vi "Measure - con-stay.vi"() -> ()   [LabVIEW 2013]
panel:
  in  "errorOutt":errorcluster
  in  "Error":bool
  in  "SetOutput":bool
  in  "NeedToSetOutput":bool
  out "Output":string
  out "SetCurrentStr":string
  out "SetVoltageStr":string
  in  "SetVoltage":dbl format="%#.3g"
  in  "SetCurrent":dbl
  in  "NeedToSetVoltage":bool
  in  "NeedToSetCurrent":bool
  in  "Active":bool
  out "connection ID":refnum<k5>
  in  "Connect":bool
  out "GetCurrent":string
  in  "Adress":string="172.16.21.19"
  out "GetVoltage":string
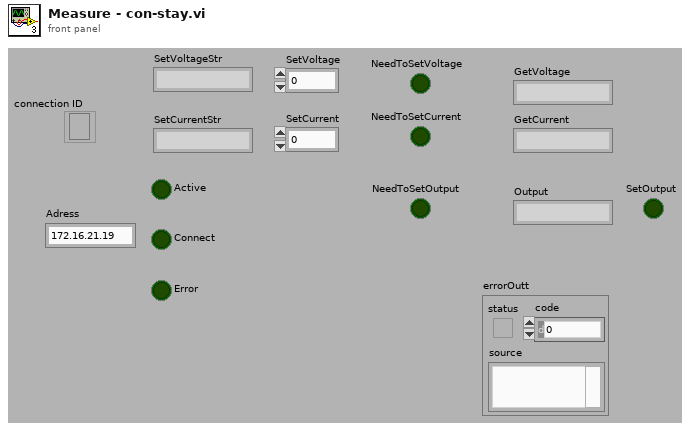
[diagram p1: front panel]
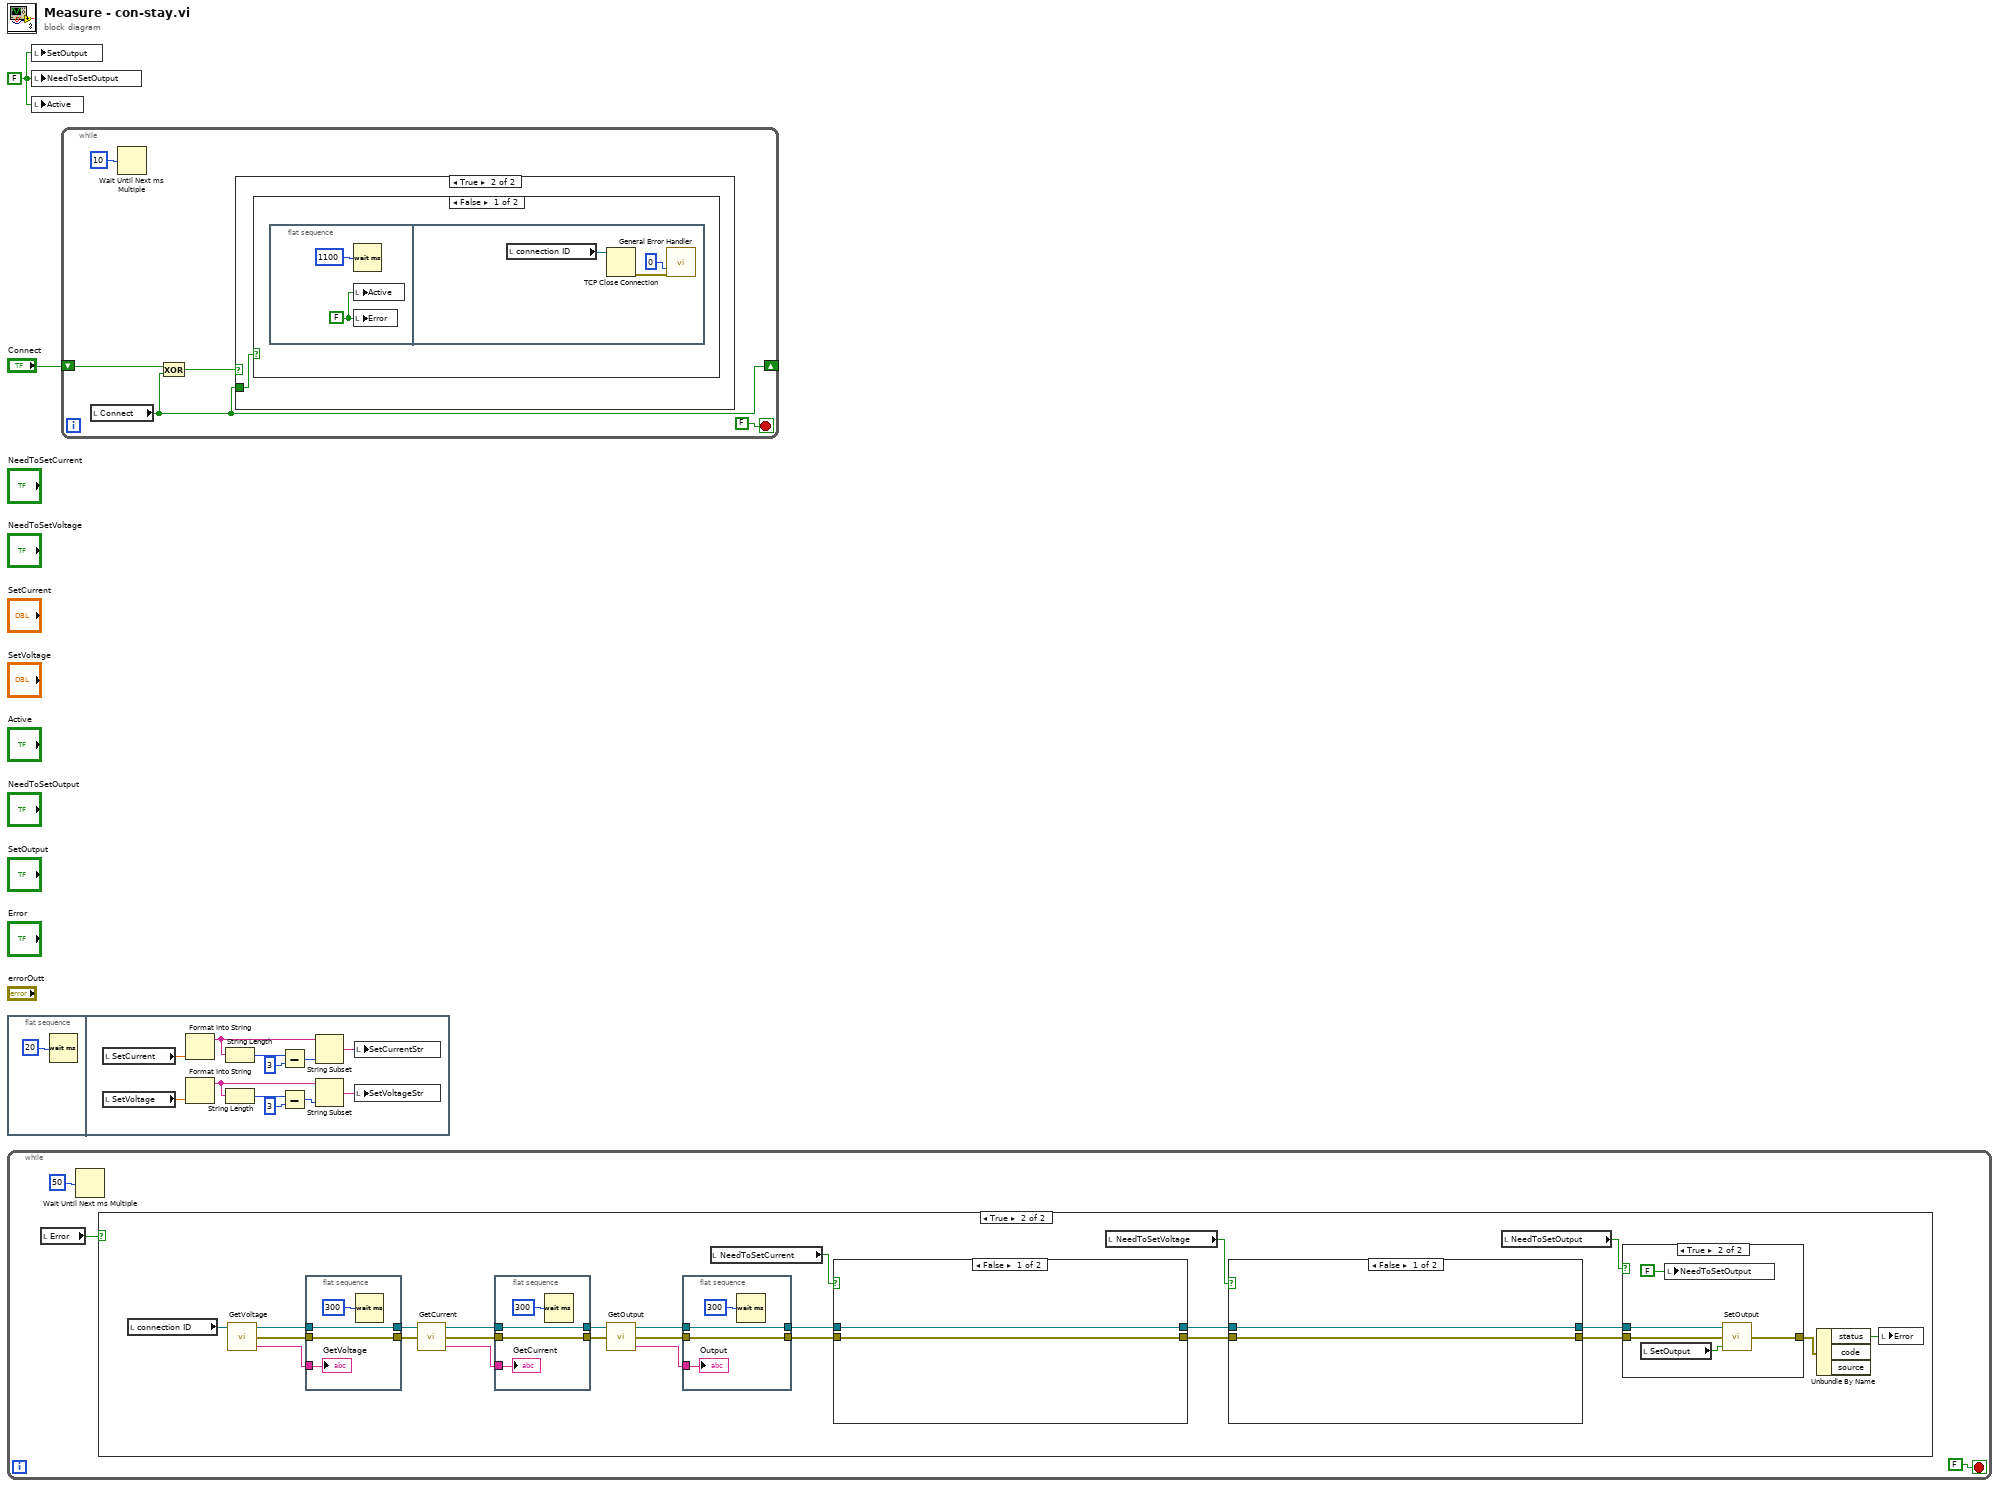
[diagram p0: block diagram]
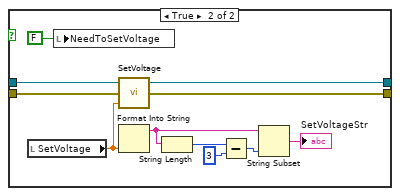
[diagram p4: hidden frame]
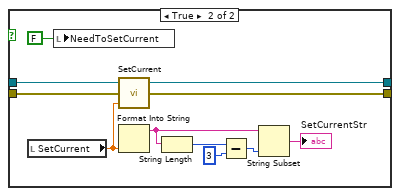
[diagram p5: hidden frame]
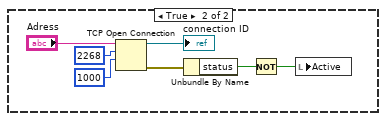
[diagram p7: hidden frame]
diagram:
  w1 = FALSE ("Active")
  n1 = flat-sequence {
    frame #0 {
      n2 = Wait (ms)(milliseconds to wait=u32 20 ("millisecond multiple")) -> ()  [unwired: 1 out]
    }
    frame #1 {
      n3 = local read "SetCurrent"() -> (w11:dbl)
      n4 = local read "SetVoltage"() -> (w10:dbl)
      n5 = Format Into String(w11) -> (resulting string=w15:string)  [unwired: 3 in, 1 out]
      n6 = Format Into String(w10) -> (resulting string=w6:string)  [unwired: 3 in, 1 out]
      n7 = String Length(string=w15) -> (length=w14:i32)
      n8 = String Length(string=w6) -> (length=w9:i32)
      n9 = Subtract(x=w14, y=3) -> (x-y=w12:i32)
      n10 = Subtract(x=w9, y=3) -> (x-y=w7:i32)
      n11 = String Subset(string=w15, length (rest)=w12) -> (substring=w4:string)  [unwired: 1 out]
      n12 = String Subset(string=w6, length (rest)=w7) -> (substring=w5:string)  [unwired: 1 out]
      n13 = local write "SetCurrentStr"(w4) -> ()
      n14 = local write "SetVoltageStr"(w5) -> ()
    }
  }
  n15 = while {
    stop <- FALSE stop-if-true
    n16 = local read "Error"() -> (w17:bool)
    n17 = Wait Until Next ms Multiple(millisecond multiple=u32 50) -> ()  [unwired: 1 out]
    n18 = case shown="True" w17 {
      frame False {
      }
      frame True {
        n19 = local read "connection ID"() -> (w43:refnum<k5>)
        n20 = call "GetVoltage.vi"("connection ID"=w43) -> ("Voltage"=w31:string, "error out"=w30:errorcluster, "connection ID out"=w33:refnum<k5>)  [unwired: 1 in, 1 out]
        n21 = flat-sequence {
          tunnel: w33 -> [w55]
          tunnel: [w55] -> w32
          tunnel: w31 -> [w54]
          tunnel: [w53] -> w29
          tunnel: w30 -> [w53]
          frame #0 {
            n22 = Wait (ms)(milliseconds to wait=u32 300) -> ()  [unwired: 1 out]
            "GetVoltage" <- w54
          }
        }
        n23 = call "GetCurrent.vi"("error in"=w29, "connection ID"=w32) -> ("Current"=w24:string, "error out"=w28:errorcluster, "connection ID out"=w25:refnum<k5>)  [unwired: 1 out]
        n24 = flat-sequence {
          tunnel: [w51] -> w27
          tunnel: w28 -> [w51]
          tunnel: w25 -> [w50]
          tunnel: [w50] -> w26
          tunnel: w24 -> [w49]
          frame #0 {
            n25 = Wait (ms)(milliseconds to wait=u32 300) -> ()  [unwired: 1 out]
            "GetCurrent" <- w49
          }
        }
        n26 = call "GetOutput.vi"("error in"=w27, "connection ID"=w26) -> ("Output"=w23:string, "error out"=w22:errorcluster, "connection ID out"=w21:refnum<k5>)  [unwired: 1 out]
        n27 = flat-sequence {
          tunnel: [w47] -> w19
          tunnel: w22 -> [w47]
          tunnel: w21 -> [w46]
          tunnel: [w46] -> w20
          tunnel: w23 -> [w44]
          frame #0 {
            n28 = Wait (ms)(milliseconds to wait=u32 300) -> ()  [unwired: 1 out]
            "Output" <- w44
          }
        }
        n29 = local read "NeedToSetCurrent"() -> (w40:bool)
        n30 = case shown="False" w40 {
          tunnel: [w75 w87] -> w42
          tunnel: [w76 w79] -> w37
          tunnel: w19 -> [w76 w78]
          tunnel: w20 -> [w75 w77]
          frame False {
          }
          frame True {
            n31 = local read "SetCurrent"() -> (w85:dbl)
            n32 = local write "NeedToSetCurrent"(FALSE ("NeedToSetCurrent")) -> ()
            n33 = call "SetCurrent.vi"("Current"=w85, "error in"=w78, "connection ID"=w77) -> ("error out"=w79:errorcluster, "connection ID out"=w87:refnum<k5>)  [unwired: 1 out]
            n34 = Format Into String(w85) -> (resulting string=w80:string)  [unwired: 3 in, 1 out]
            n35 = String Length(string=w80) -> (length=w82:i32)
            n36 = Subtract(x=w82, y=3) -> (x-y=w84:i32)
            n37 = String Subset(string=w80, length (rest)=w84) -> (substring=→"SetCurrentStr":string)  [unwired: 1 out]
          }
        }
        n38 = local read "NeedToSetVoltage"() -> (w41:bool)
        n39 = case shown="False" w41 {
          tunnel: w42 -> [w63 w74]
          tunnel: [w63 w66] -> w39
          tunnel: w37 -> [w62 w65]
          tunnel: [w62 w64] -> w36
          frame False {
          }
          frame True {
            n40 = local read "SetVoltage"() -> (w72:dbl)
            n41 = local write "NeedToSetVoltage"(FALSE ("NeedToSetVoltage")) -> ()
            n42 = call "SetVoltage.vi"("Voltage"=w72, "error in"=w65, "connection ID"=w74) -> ("error out"=w64:errorcluster, "connection ID out"=w66:refnum<k5>)  [unwired: 1 out]
            n43 = Format Into String(w72) -> (resulting string=w68:string)  [unwired: 3 in, 1 out]
            n44 = String Length(string=w68) -> (length=w71:i32)
            n45 = Subtract(x=w71, y=3) -> (x-y=w69:i32)
            n46 = String Subset(string=w68, length (rest)=w69) -> (substring=→"SetVoltageStr":string)  [unwired: 1 out]
          }
        }
        n47 = local read "NeedToSetOutput"() -> (w38:bool)
        n48 = case shown="True" w38 {
          tunnel: w39 -> [_ w59]
          tunnel: w36 -> [w56 w58]
          tunnel: [w56 w57] -> w35
          frame False {
          }
          frame True {
            n49 = local read "SetOutput"() -> (w60:bool)
            n50 = local write "NeedToSetOutput"(FALSE ("NeedToSetVoltage")) -> ()
            n51 = call "SetOutput.vi"("State"=w60, "error in"=w58, "connection ID"=w59) -> ("error out"=w57:errorcluster)  [unwired: 2 out]
          }
        }
        n52 = Unbundle By Name(w35) -> ("status"=w34:bool)  [unwired: 2 out]
        n53 = local write "Error"(w34) -> ()
      }
    }
  }
  n54 = local write "SetOutput"(w1) -> ()
  n55 = local write "NeedToSetOutput"(w1) -> ()
  n56 = local write "Active"(w1) -> ()
  n57 = while {
    shift-right: [w89] -> _
    shift-left: "Connect" -> [w90]
    stop <- FALSE stop-if-true
    n58 = local read "Connect"() -> (w89:bool)
    n59 = Wait Until Next ms Multiple(millisecond multiple=u32 10) -> ()  [unwired: 1 out]
    n60 = Exclusive Or(1:w89, 2:w90) -> (0:w91:bool)
    n61 = case shown="True" w91 {
      tunnel: w89 -> [_ w93]
      frame False {
      }
      frame True {
        n62 = case shown="False" w93 {
          frame False {
            n63 = flat-sequence {
              frame #0 {
                w95 = FALSE ("Active")
                n64 = Wait (ms)(milliseconds to wait=u32 1100 ("millisecond multiple")) -> ()  [unwired: 1 out]
                n65 = local write "Active"(w95) -> ()
                n66 = local write "Error"(w95) -> ()
              }
              frame #1 {
                n67 = local read "connection ID"() -> (w98:refnum<k5>)
                n68 = TCP Close Connection(connection ID=w98) -> (error out=w97:errorcluster)  [unwired: 1 in, 2 out]
                n69 = call <vilib>:"General Error Handler.vi"("type of dialog (OK msg:1)"=u32 0 ("millisecond multiple"), "error in (no error)"=w97) -> ()  [unwired: 9 in, 5 out]
              }
            }
          }
          frame True {
            n70 = TCP Open Connection(address="Adress", remote port or service name=u16 2268 ("Port"), timeout ms (60000)=1000) -> (connection ID=→"connection ID":refnum<k5>, error out=w105:errorcluster)  [unwired: 1 in, 1 out]
            n71 = Unbundle By Name(w105) -> ("status"=w100:bool)
            n72 = Not(x=w100) -> (.not. x?=w99:bool)
            n73 = local write "Active"(w99) -> ()
          }
        }
      }
    }
  }
